vi "motoresstartstop.vi"(0 "NXTIN":T1) -> (1 "NXT OUT":T1, 2 "FinalizarPrograma?":bool)   [LabVIEW 2012, in "ExemploFinal.lvrbt"]
uses:
  ExemploFinal.lvrbt
  <vilib>/NXT/Subs/LVHSConnector.ctl
  <vilib>/NXT/LegoClasses/BrickReference/BrickReference.lvclass
  <vilib>/NXT/Subs/MotorOutput.ctl
panel:
  # "Este VI controla os motores de movimento do TRIBOT de acordo com aos valores obtidos dos sensores.\nCaso uma das opções abaixo ocorra os motores de movimento são desligados:\n   -Sensor Touch pressionado\n   - Sensor de Ruído detecta valores acima de 30%\n   - Sensor de Luz detecta iluminação maior que 50%\n   - Sensor Ultrasônico detecta uma distânica menor que 10cm\nSe o sensor Ultrasônico detectar uma distância menor que 50cm os motores diminuem a velocidade de acordo com a distância encontrada."
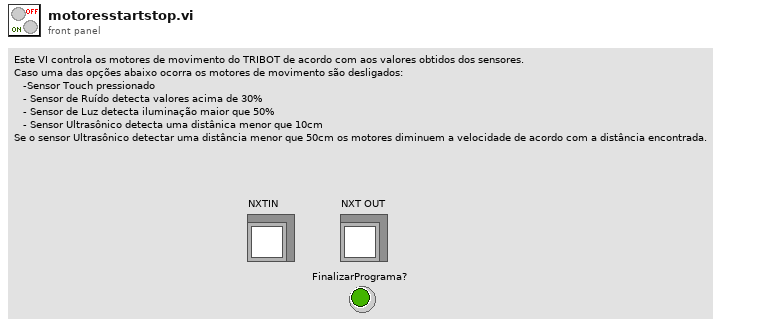
[diagram p1: front panel]
types:
  T1 = typedef "LVHSConnector.ctl" = refnum<class "BrickReference.lvclass">
  T2 = typedef "MotorOutput.ctl" = u8
  T3 = cluster{"TouchOUT":bool, "SomOUT":i32, "LuzOUT":i32, "UltrasomOUT":i32, "BotãoOUT":bool}
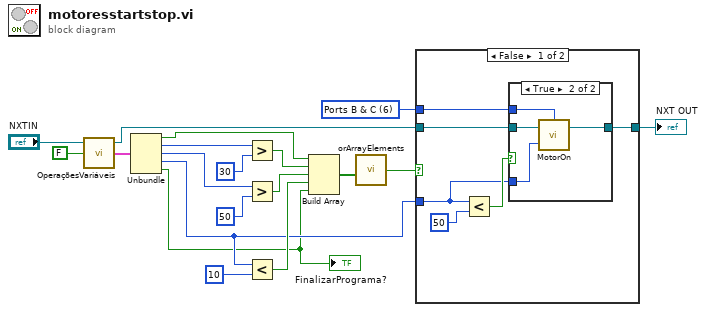
[diagram p0: block diagram]
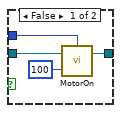
[diagram p2: hidden frame]
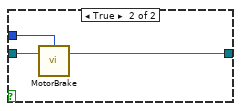
[diagram p3: hidden frame]
diagram:
  w12 = T2 6 items=["Port A"=0, "Port B"=1, "Port C"=2, "Ports A & B"=4, "Ports A & C"=5, "Ports B & C"=6, "All Ports"=3] ("Port (All Ports)")
  n1 = call "OperaçõesVariáveis.vi"("Escrever?"=FALSE, "NXT IN"="NXTIN") -> ("Saídas"=w10:T3, "NXT OUT"=w1:T1)  [unwired: 1 in, 1 out]
  n2 = Unbundle(w10) -> ("TouchOUT"=w9:bool, "SomOUT"=w8:i32, "LuzOUT"=w7:i32, "UltrasomOUT"=w6:i32, "BotãoOUT"=w3:bool)
  "FinalizarPrograma?" <- w3
  n3 = Greater?(x=w8, y=30) -> (0:w19:bool)
  n4 = Greater?(x=w7, y=50) -> (0:w18:bool)
  n5 = Less?(x=w6, y=10) -> (x < y?=w17:bool)
  n6 = Build Array(w9, w19, w18, w17, w3) -> (w16:bool[])
  n7 = call <vilib>:"orArrayElements.vi"("Boolean Array"=w16) -> ("Logical OR"=w15:bool)
  n8 = case shown="False" w15 {
    tunnel: w12 -> [w22 w36]
    tunnel: w6 -> [w23 _]
    tunnel: [w21 w35] -> w2
    tunnel: w1 -> [w20 w34]
    frame False {
      n9 = Less?(x=w23, y=50) -> (x < y?=w24:bool)
      n10 = case shown="True" w24 {
        tunnel: w23 -> [_ w33]
        tunnel: w22 -> [w29 w32]
        tunnel: [w27 w31] -> w21
        tunnel: w20 -> [w26 w30]
        frame False {
          n11 = call <vilib>:"MotorOn.vi"("Power (75)"=100, "NXT/EV3"=w26, "Output Port (All Ports)"=w29) -> ("NXT/EV3"=w27:T1)  [unwired: 1 in]
        }
        frame True {
          n12 = call <vilib>:"MotorOn.vi"("Power (75)"=w33, "NXT/EV3"=w30, "Output Port (All Ports)"=w32) -> ("NXT/EV3"=w31:T1)  [unwired: 1 in]
        }
      }
    }
    frame True {
      n13 = call <vilib>:"MotorBrake.vi"("NXT/EV3"=w34, "Port (All Ports)"=w36) -> ("NXT/EV3"=w35:T1)  [unwired: 2 in]
    }
  }
  "NXT OUT" <- w2
